vi "set gobject size.vi"(8 "error in":errorcluster, 10 "size":T1, 11 "object refnum":refnum<vi>) -> (0 "error out":errorcluster)   [LabVIEW 2013, in "PL Framework Configuration Tool.lvlib" / "EngineTags.lvclass"]
uses:
  EngineTags.lvclass
  <vilib>/Utility/miscctls.llb/LVBoundsTypeDef.ctl
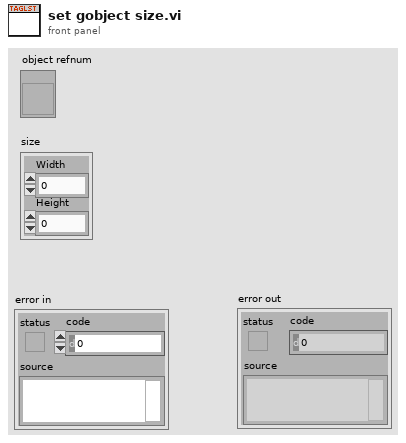
[diagram p1: front panel]
types:
  T1 = typedef "LVBoundsTypeDef.ctl" = cluster{"Width":u32, "Height":u32}
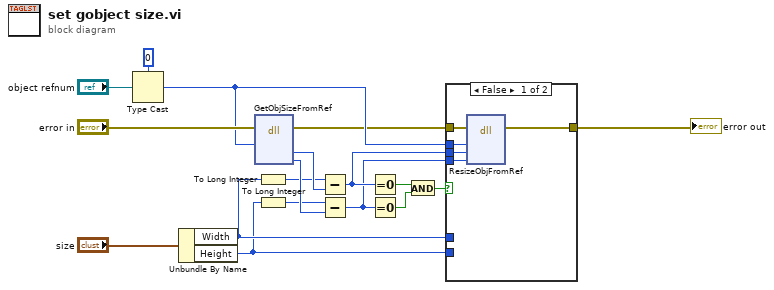
[diagram p0: block diagram]
diagram:
  n1 = Type Cast(type=0, x="object refnum") -> (*(type *) &x=w13:i32)
  n2 = Unbundle By Name("size") -> ("Width"=w2:u32, "Height"=w1:u32)
  n3 = dll-call lib="LabVIEW" fn="GetObjSizeFromRef"(error in="error in", "objRef"=w13) -> (error out=w12:errorcluster, "width"=w11:i32, "height"=w10:i32)  [unwired: 6 in, 1 out]
  n4 = To Long Integer(number=w2) -> (32bit integer=w9:i32)
  n5 = To Long Integer(number=w1) -> (32bit integer=w8:i32)
  n6 = Subtract(x=w9, y=w11) -> (x-y=w7:i32)
  n7 = Subtract(x=w8, y=w10) -> (x-y=w6:i32)
  n8 = Equal To 0?(x=w7) -> (x = 0?=w4:bool)
  n9 = Equal To 0?(x=w6) -> (x = 0?=w5:bool)
  n10 = And(x=w4, y=w5) -> (x .and. y?=w3:bool)
  n11 = case shown="False" w3 {
    tunnel: w12 -> [w23 w24]
    tunnel: w13 -> [w22 _]
    tunnel: [w21 w24] -> w17
    tunnel: w7 -> [w20 _]
    tunnel: w6 -> [w19 _]
    tunnel: w2 -> [_ _]
    tunnel: w1 -> [_ _]
    frame False {
      n12 = dll-call lib="LabVIEW" fn="ResizeObjFromRef"(error in=w23, "ref"=w22, "deltaHoriz"=w20, "deltaVert"=w19) -> (error out=w21:errorcluster)  [unwired: 6 in, 1 out]
    }
    frame True {
    }
  }
  "error out" <- w17
